vi "Merge.vi"(2 "Keyed Array In 2":T1, 3 "Keyed Array In 1":T1) -> (0 "Merged Keyed Array":T1)   [LabVIEW 2012, in "TLB` Template.lvlib" / "Tools_KeyedArray.lvlib"]
uses:
  Tools_KeyedArray.lvlib
  KeyedArray.ctl
  Map String.vi
  String/Get Case Matching.vi
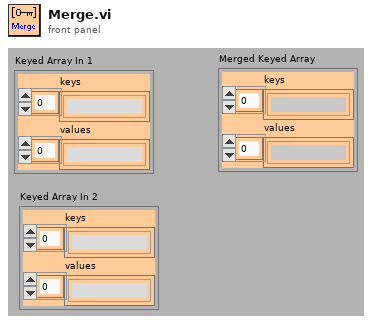
[diagram p1: front panel]
types:
  T1 = typedef "TLB` Template.lvlib/Tools_KeyedArray.lvlib/KeyedArray.ctl" = cluster{"keys":string[], "values":string[]}
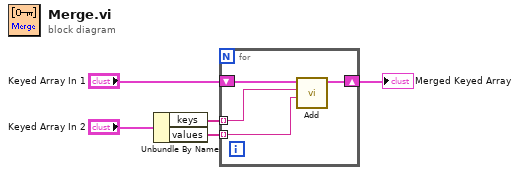
[diagram p0: block diagram]
diagram:
  n1 = Unbundle By Name("Keyed Array In 2") -> ("keys"=w3:string[], "values"=w2:string[])
  n2 = for {
    shift-right: [w8] -> w1
    shift-left: "Keyed Array In 1" -> [w9]
    tunnel: w3 -> [w7] mode=indexing
    tunnel: w2 -> [w6] mode=indexing
    n3 = call "Add.vi"("value"=w6, "key"=w7, "array in"=w9) -> ("array out"=w8:T1)  [unwired: 1 in, 3 out]
  }
  "Merged Keyed Array" <- w1
